vi "set_request_body_form.vi"(8 "error in":errorcluster, 9 "value":string, 10 "key":string, 11 "obj in":refnum<class "RequestBuilder.lvclass">) -> (0 "error out":errorcluster, 2 "success":bool, 3 "obj out":refnum<class "RequestBuilder.lvclass">)   [LabVIEW 2020, in "reqwest.lvlib" / "RequestBuilder.lvclass"]
doc: "Use this to submit simple key-value data (like login credentials, search parameters, or form fields) to web services that expect HTML form-style data - it automatically sets the Content-Type: application/x-www-form-urlencoded header and call it multiple times to build up all your form fields."
uses:
  RequestBuilder.lvclass
  RequestBuilder.lvclass/RequestBuilder.ctl
  lv_reqwest_64.dll
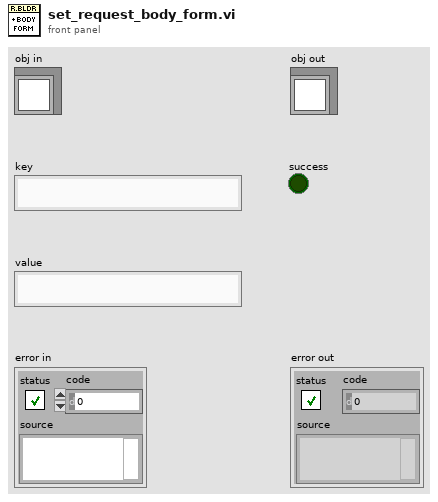
[diagram p1: front panel]
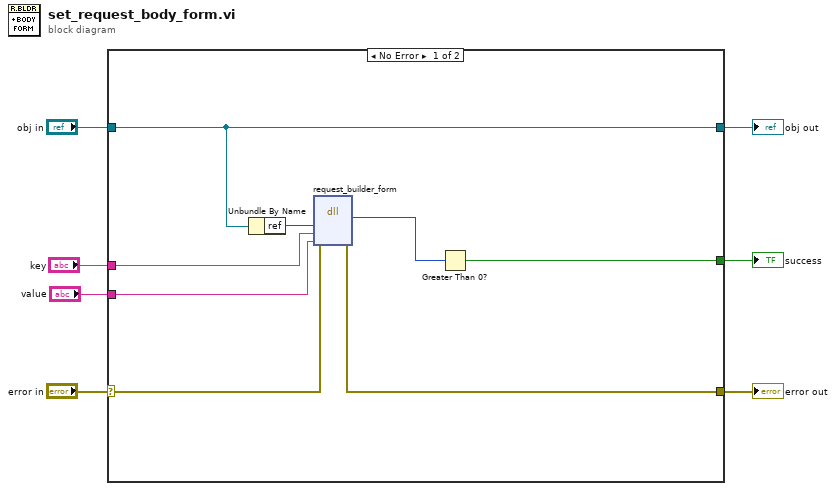
[diagram p0: block diagram]
diagram:
  n1 = case shown="No Error" "error in" {
    selector: "error in" -> [w15 w17]
    tunnel: "obj in" -> [w14 w16]
    tunnel: [w9 w17] -> w5
    tunnel: [w14 w16] -> w4
    tunnel: "key" -> [w12 _]
    tunnel: [w10 _] -> w2
    tunnel: "value" -> [w8 _]
    frame No Error {
      n2 = Unbundle By Name(w14) -> ("ref"=w13:u64)
      n3 = dll-call lib="C:/code/reqwest-rs-labview/lv_src/lv_reqwest_*.*" fn="request_builder_form"(error in=w15, "builder_ptr"=w13, "key"=w12, "value"=w8) -> (error out=w9:errorcluster, "Return Value"=w11:u8)  [unwired: 5 in, 1 out]
      n4 = Greater Than 0?(x=w11) -> (x > 0?=w10:bool)
    }
    frame Error {
    }
  }
  "error out" <- w5
  "obj out" <- w4
  "success" <- w2
